vi "FGV.vi"(7 "Method (Get)":enum16{"Get", "Set"}(ring), 8 "error in":errorcluster, 10 "Data In":variant, 11 "Name":T1) -> (0 "error out":errorcluster, 3 "Data out":variant)   [LabVIEW 2021]
uses:
  Controls/Measure Type.ctl
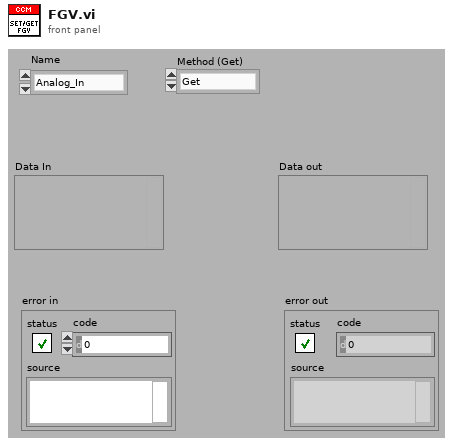
[diagram p1: front panel]
types:
  T1 = typedef "Measure Type.ctl" = enum16{"Analog_In", "Analog_Out", "Digital_In", "Digital_Out", "Switch", "NI_DMM"}
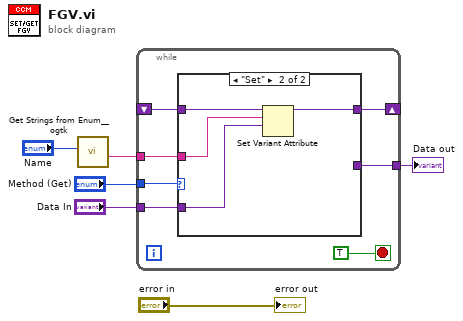
[diagram p0: block diagram]
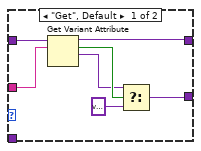
[diagram p2: hidden frame]
diagram:
  n1 = call <userlib>:"Get Strings from Enum__ogtk.vi"("Enum"="Name") -> ("String Value"=w1:string)  [unwired: 7 in, 3 out]
  n2 = while {
    tunnel: "Method (Get)" -> [w13]
    tunnel: w1 -> [w10]
    shift-right: [w11] -> _
    shift-left: _ -> [w12]
    tunnel: [w8] -> w3
    tunnel: "Data In" -> [w7]
    stop <- TRUE stop-if-true
    n3 = case shown="\"Set\"" w13 {
      tunnel: w7 -> [_ w21]
      tunnel: w12 -> [w20 w24]
      tunnel: [w19 w23] -> w11
      tunnel: w10 -> [w18 w22]
      tunnel: [w15 _] -> w8
      frame "Get", Default {
        n4 = Get Variant Attribute(Variant=w20, name=w18) -> (duplicate Variant=w19:variant, found=w17:bool, value=w16:variant)  [unwired: 2 in, 1 out]
        n5 = Select(t=w16, s=w17, f=variant) -> (s? t:f=w15:variant)
      }
      frame "Set" {
        n6 = Set Variant Attribute(Variant=w24, name=w22, value=w21) -> (Variant out=w23:variant)  [unwired: 1 in, 2 out]
      }
    }
  }
  "Data out" <- w3
  "error out" <- "error in"
